vi "Analog Output (Host).vi"(0 "RIO Device":T1="RIO0::INSTR") -> ()   [LabVIEW 2012]
doc: "This VI will will initialize the FPGA VI and then continually write single point values to 4 channels."
uses:
  <vilib>/Utility/error.llb/DialogType.ctl
  <vilib>/rvi/interface/nirviReadWriteControl/nirviReadWriteControl.xnode
  <vilib>/rvi/interface/nirviCloseFPGA/nirviCloseFPGA.xnode
  <vilib>/rvi/interface/nirviOpenFPGA/nirviOpenFPGA.xnode
  Analog Output (FPGA).vi
  FPGA Bitfiles/AnalogOutput-RSe_FPGATarget2_AnalogOutput(FPG_CKYJr+NdypY.lvbitx
  <vilib>/FPGAPlugInAG/PCIe-7851R/niLvFpga_Open_PCIe-7851R.vi
  NiFpgaLv.dll
  <vilib>/Utility/error.llb/Error Cluster From Error Code.vi
  <vilib>/rvi/errors/niLvFpgaAdjustHostInterfaceError.vi
  <vilib>/FPGAPlugInAG/PCIe-7851R/niLvFpga_Close_PCIe-7851R.vi
  <vilib>/userdefined/High Color/nirio_resource_hc.ctl
panel:
  in  "stop 2":bool
  out "FPGA Error?":bool
  out "FPGA Error Message":string
  in  "AO3 (V)":dbl(knob) scale=-10.0..10.0
  in  "AO2 (V)":dbl(knob) scale=-10.0..10.0
  in  "AO1 (V)":dbl(knob) scale=-10.0..10.0
  in  "AO0 (V)":dbl(knob) scale=-10.0..10.0
  # "Analog Output"
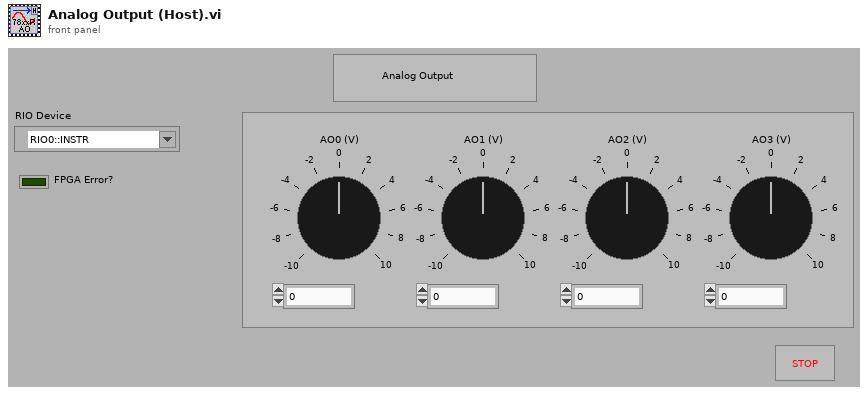
[diagram p1: front panel]
types:
  T1 = typedef "nirio_resource_hc.ctl" = tag
  T2 = typedef "DialogType.ctl" = u16
  T3 = cluster{"[0]":i16, "[1]":i16, "[2]":i16, "[3]":i16}
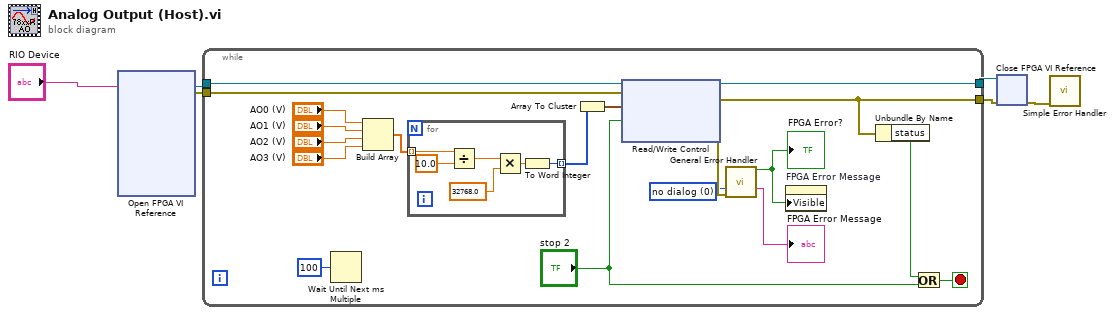
[diagram p0: block diagram]
diagram:
  n1 = xnode "Open FPGA VI Reference"("resource name"="RIO Device") -> ("FPGA VI Reference Out"=w2:refnum<k20>, "error out"=w1:errorcluster)  [unwired: 1 in]
  n2 = while {
    tunnel: w2 -> [w24]
    tunnel: [w25] -> w6
    tunnel: w1 -> [w21]
    tunnel: [w12] -> w5
    stop <- w9 stop-if-true
    w8 = T2 0 items=["no dialog", "OK message", "continue or stop message", "OK message + warnings", "continue/stop + warnings"] ("type of dialog (OK msg:1)")
    n3 = Wait Until Next ms Multiple(millisecond multiple=u32 100) -> ()  [unwired: 1 out]
    n4 = Build Array("AO0 (V)", "AO1 (V)", "AO2 (V)", "AO3 (V)") -> (w13:dbl[])
    n5 = for {
      tunnel: [w26] -> w22 mode=indexing
      tunnel: w13 -> [w31] mode=indexing
      n6 = Divide(x=w31, y=10.0) -> (x/y=w29:dbl)
      n7 = Multiply(x=w29, y=32768.0) -> (x*y=w27:dbl)
      n8 = To Word Integer(number=w27) -> (16bit integer=w26:i16)
    }
    n9 = Array To Cluster(array=w22) -> (cluster=w23:T3)
    n10 = xnode "Read/Write Control"("FPGA VI Reference In"=w24, "error in"=w21, "AO Data"=w23, "stop"="stop 2") -> ("FPGA VI Reference Out"=w25:refnum<k20>, "error out"=w12:errorcluster, "FPGA Error Out"=w20:errorcluster)
    n11 = call <vilib>:"General Error Handler.vi"("type of dialog (OK msg:1)"=w8, "error in (no error)"=w20) -> ("error?"=w18:bool, "message"=→"FPGA Error Message":string)  [unwired: 9 in, 3 out]
    "FPGA Error?" <- w18
    n12 = property on="FPGA Error Message" class="Str"("Visible"=w18) -> ()  [unwired: 2 in, 2 out]
    n13 = Unbundle By Name(w12) -> ("status"=w11:bool)
    n14 = Or(x=w11, y="stop 2") -> (x .or. y?=w9:bool)
  }
  n15 = xnode "Close FPGA VI Reference"("FPGA VI Reference In"=w6, "error in"=w5) -> ("error out"=w4:errorcluster)
  n16 = call <vilib>:"Simple Error Handler.vi"("error in (no error)"=w4) -> ()  [unwired: 4 in, 5 out]
